vi "GetID.vi"(8 "error in (no error)":errorcluster, 11 "Appender in":refnum<class "Appender.lvclass">) -> (0 "error out":errorcluster, 2 "ID":string, 3 "Appender out":refnum<class "Appender.lvclass">)   [LabVIEW 2026, in "Lumberjack.lvlib" / "Appender.lvclass"]
doc: "Apply this appender's acceptance logic to one Statement. First the per-appender threshold: compare the statement's level against config.threshold by rank (RankCompare), rejecting anything below threshold. Then the Filter: mirror accepts everything that passed the threshold; routed accepts only statements whose level is within the inclusive rank band [levelMin, levelMax] and whose sourceTag matches tagPrefix (empty prefix matches any; a non-empty prefix matches on a dot-hierarchy boundary, so app.db matches app.db and app.db.query but not app.database). On acceptance, call the dynamic-dispatch Write with the Statement; on rejection, do nothing. Does not format (Write does) and does not enforce queue backpressure (that is the Actor Core intake path). Static; protected (SRS-LMBR-009, 026, 027)."
uses:
  Appender.lvclass
  Appender.lvclass/Appender.ctl
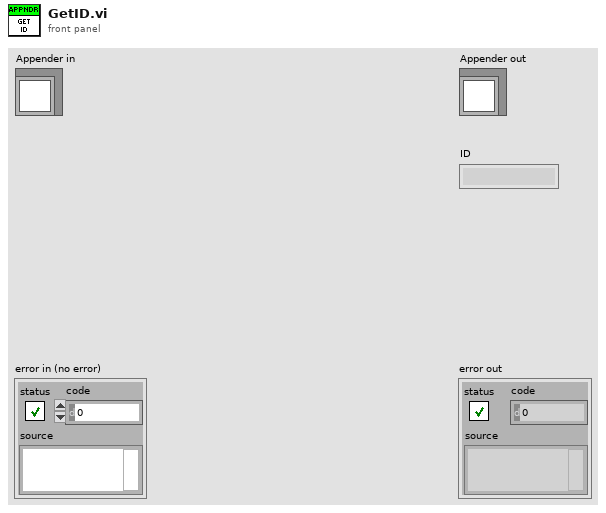
[diagram p1: front panel]
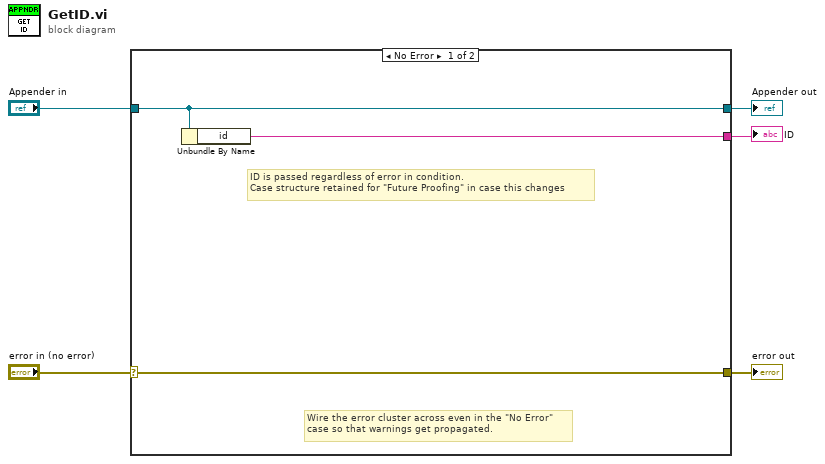
[diagram p0: block diagram]
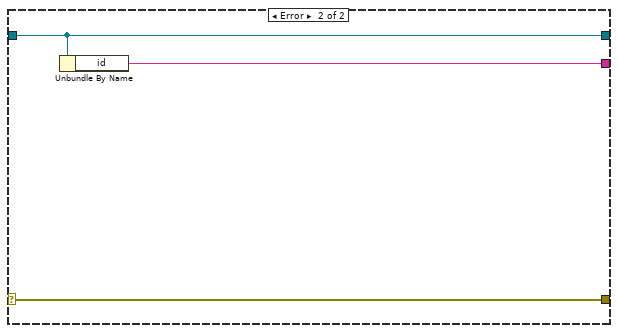
[diagram p2: hidden frame]
diagram:
  n1 = case shown="No Error" "error in (no error)" {
    selector: "error in (no error)" -> [w8 w11]
    tunnel: [w8 w11] -> w4
    tunnel: [w7 w9] -> w2
    tunnel: "Appender in" -> [w7 w9]
    tunnel: [w6 w10] -> w1
    frame No Error {
      # "ID is passed regardless of error in condition.\nCase structure retained for \"Future Proofing\" in case this changes"
      # "Wire the error cluster across even in the \"No Error\"\ncase so that warnings get propagated."
      n2 = Unbundle By Name(w7) -> ("id"=w6:string)
    }
    frame Error {
      n3 = Unbundle By Name(w9) -> ("id"=w10:string)
    }
  }
  "error out" <- w4
  "Appender out" <- w2
  "ID" <- w1
